vi "TB-Get Data Folder.vi"(0 "ID":string, 7 "Drive":string, 11 "error in (no error)":errorcluster) -> (6 "Data folder":path, 15 "error out":errorcluster)   [LabVIEW 2020]
doc: "Takes an experiment ID (e.g. KEH999) and returns the standard data folder (e.g. C:\\Data\\KEH DATA\\KEH999)"
uses:
  <vilib>/regexp/Match Regular Expression.xnode
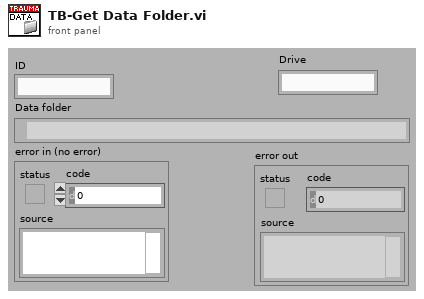
[diagram p1: front panel]
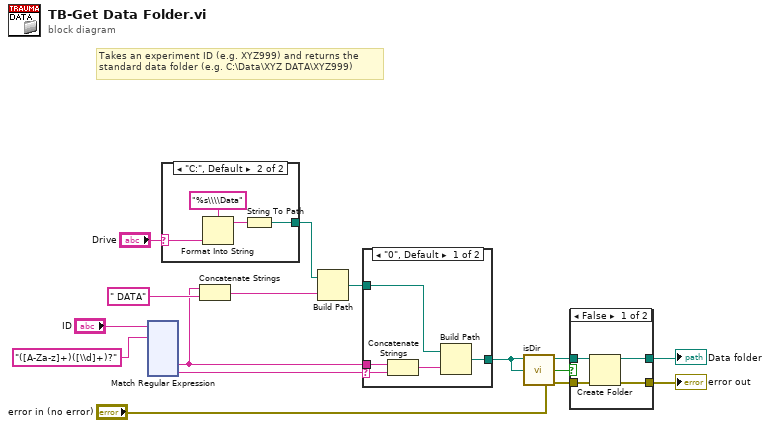
[diagram p0: block diagram]
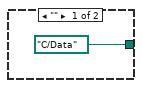
[diagram p2: hidden frame]
diagram:
  # "Takes an experiment ID (e.g. XYZ999) and returns the\nstandard data folder (e.g. C:\\Data\\XYZ DATA\\XYZ999)"
  n1 = xnode "Match Regular Expression"("input string"="ID", "regular expression"="([A-Za-z]+)([\\d]+)?") -> ("submatch 1"=w4:string, "submatch 2"=w3:string)  [unwired: 4 in, 5 out]
  n2 = case shown="\"C:\", Default" "Drive" {
    selector: "Drive" -> [_ w18]
    tunnel: [path "C:/Data" ("base path") w16] -> w8
    frame "" {
    }
    frame "C:", Default {
      n3 = Format Into String(format string="%s\\\\Data", w18) -> (resulting string=w17:string)  [unwired: 2 in, 1 out]
      n4 = String To Path(string=w17) -> (path=w16:path)
    }
  }
  n5 = Concatenate Strings(w4, " DATA" ("string")) -> (w13:string)
  n6 = Build Path(base path=w8, name or relative path=w13) -> (appended path=w2:path)
  n7 = case shown="\"0\", Default" w3 {
    selector: w3 -> [w23 _]
    tunnel: w4 -> [w24 _]
    tunnel: w2 -> [w21 w25]
    tunnel: [w20 w25] -> w1
    frame "0", Default {
      n8 = Concatenate Strings(w24, w23) -> (w22:string)
      n9 = Build Path(base path=w21, name or relative path=w22) -> (appended path=w20:path)
    }
    frame "" {
    }
  }
  n10 = call "isDir.vi"("path"=w1) -> ("is Dir?"=w5:bool)
  n11 = case shown="False" w5 {
    tunnel: w1 -> [w29 w31]
    tunnel: "error in (no error)" -> [w28 w30]
    tunnel: [w27 w31] -> w11
    tunnel: [w26 w30] -> w10
    frame False {
      n12 = Create Folder(path (use dialog)=w29, error in=w28) -> (created path=w27:path, error out=w26:errorcluster)  [unwired: 1 in, 1 out]
    }
    frame True {
    }
  }
  "Data folder" <- w11
  "error out" <- w10
